vi "Exporting.vi"() -> ()   [LabVIEW 2010]
uses:
  C:/BaseI/CodeBase/Applications/Assemblies/Spiricon.BeamGage.Automation.Interfaces.dll
  Applications/Assemblies/Spiricon.BeamGage.Automation.Interfaces.dll
  C:/BaseI/CodeBase/Applications/Assemblies/Spiricon.BeamGage.Automation.dll
  Applications/Assemblies/Spiricon.BeamGage.Automation.dll
panel:
  out "event callback refnum":refnum<k27>
  in  "FramesPerSec":dbl
  in  "FrameBuffer":dbl
  out "2D Picture":picture
  out "Callback2Exists":bool
  out "Callback1Exists":bool
  in  "STOP SERVER":bool
  in  "START_STOP":bool
  out "AExportStatusEnum":T1(ring)
  in  "EXPORT IMAGE":bool
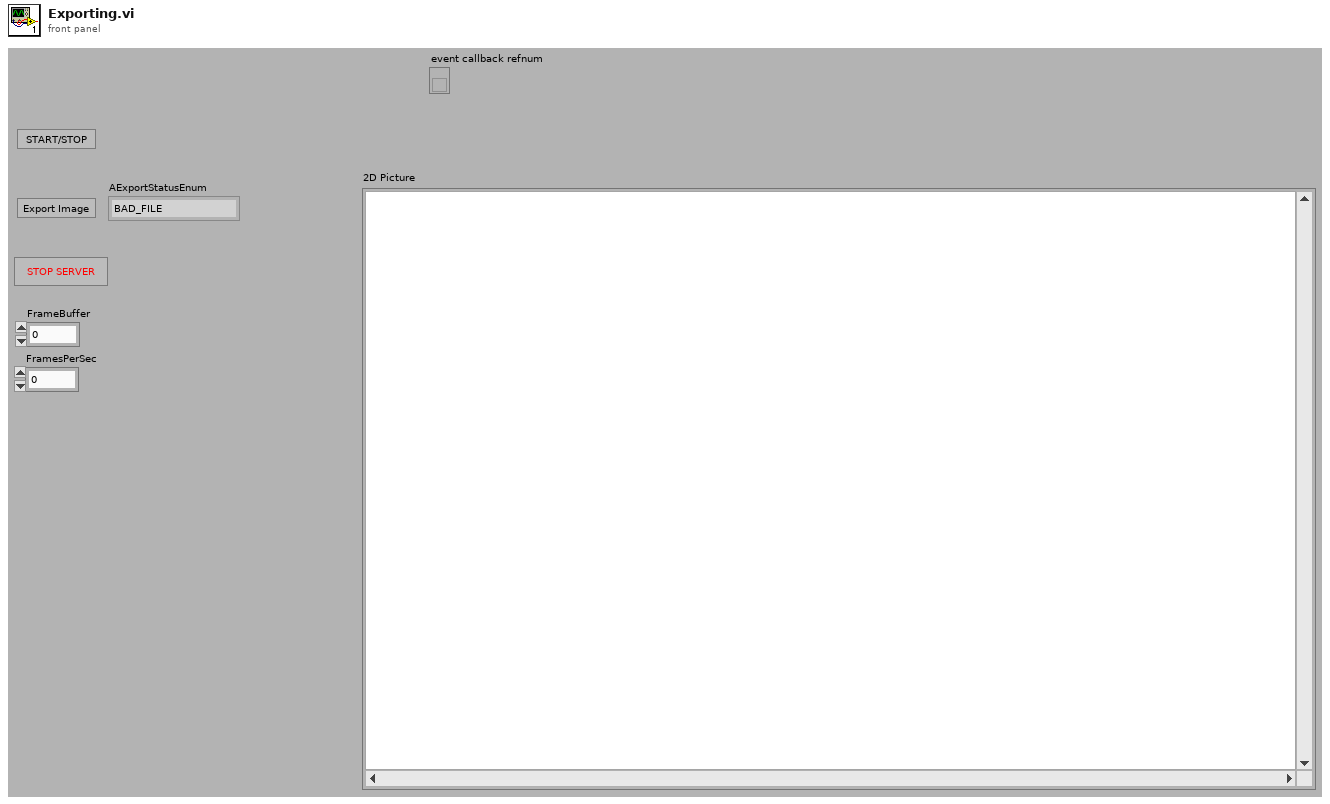
[diagram p1: front panel]
types:
  T1 = enum16{"BAD_FILE", "BAD_FRAME_NUM", "BASE_FILE_EXISTS", "BASE_FILE_IS_DIRECTORY", "GOOD", "NO_FILE_NAME", "NO_IMAGE", "READ_ONLY", "null"}
  T2 = cluster{"FrameBuffer":refnum<vi>, "2D Picture":refnum<vi>, "GetV5Instance":refnum<k24>, "FramesPerSec":refnum<vi>}
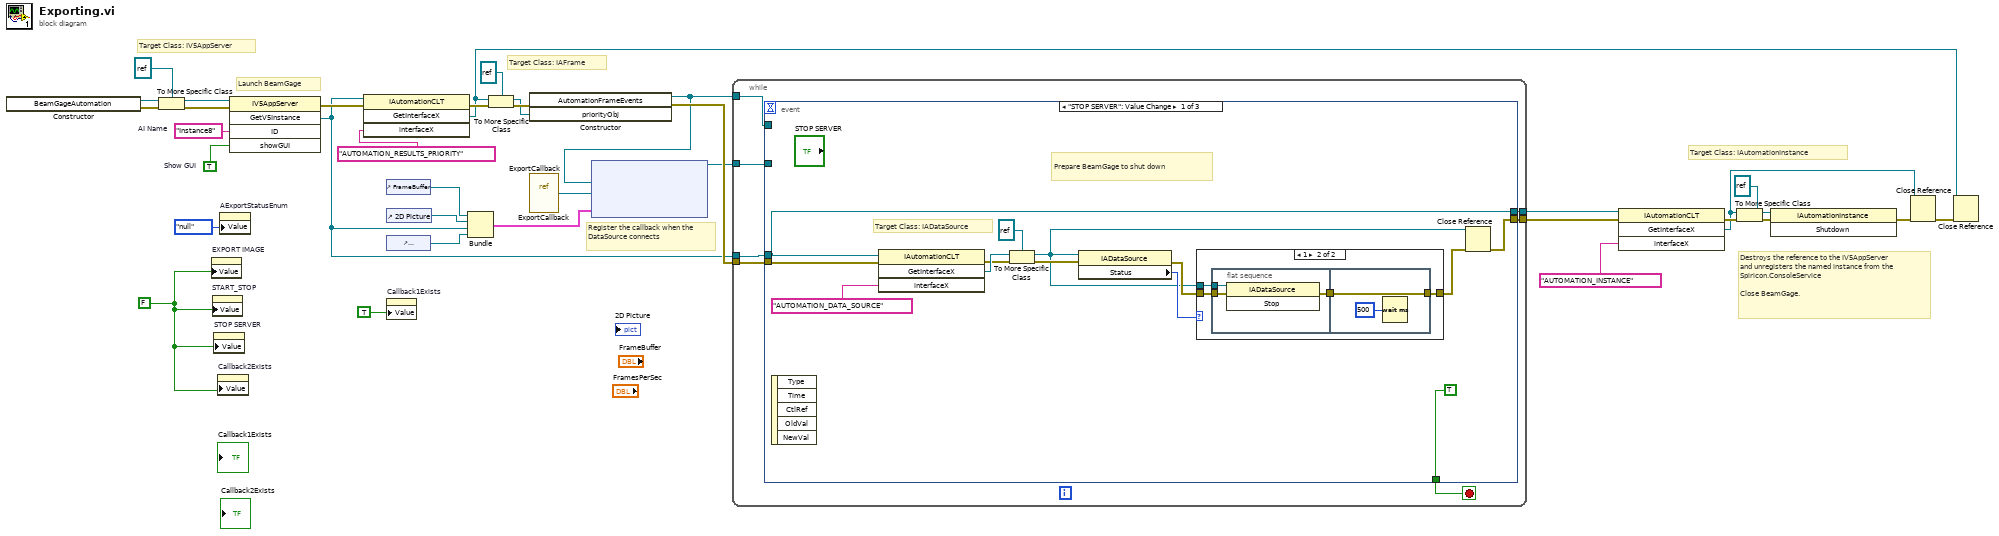
[diagram p0: block diagram]
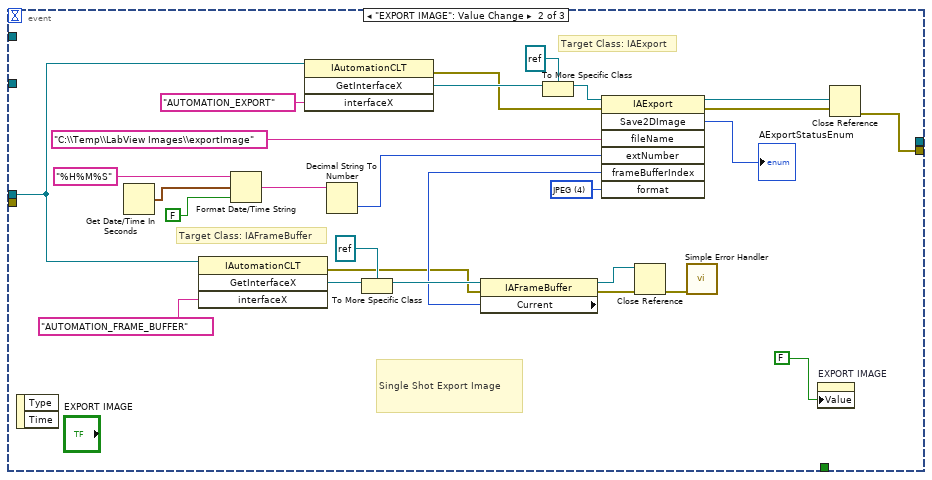
[diagram p3: hidden frame]
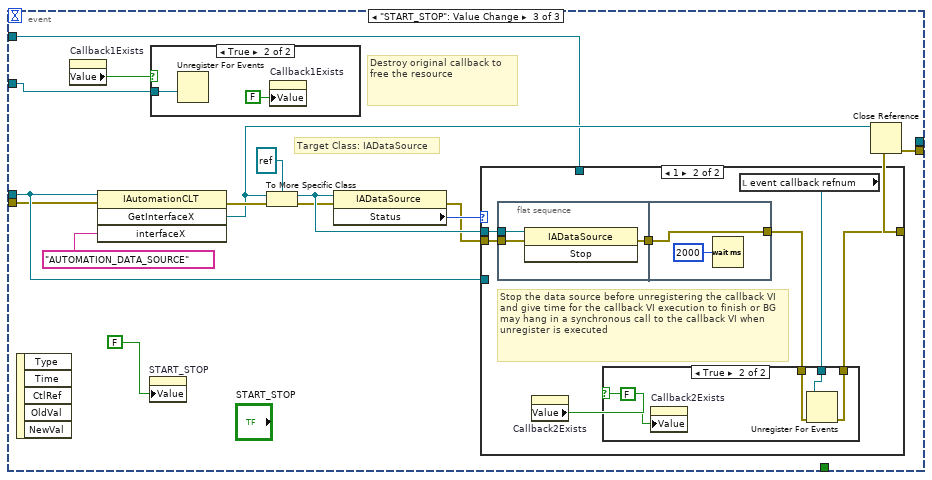
[diagram p4: hidden frame]
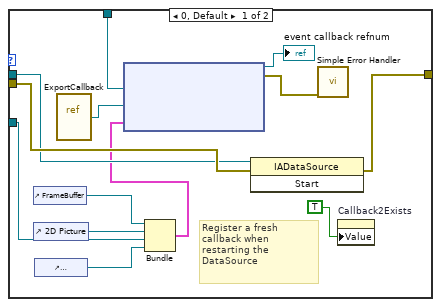
[diagram p6: hidden frame]
diagram:
  w24 = TRUE  # Show GUI
  w28 = "Instance8"  # AI Name
  w9 = FALSE ("stop")
  # "Register the callback when the DataSource connects"
  # "Launch BeamGage"
  # "Target Class: IAFrame"
  # "Target Class: IV5AppServer"
  # "Destroys the reference to the IV5AppServer and unregisters the named instance from the Spiricon.ConsoleService\n\nClose BeamGage."
  # "Target Class: IAutomationInstance"
  n1 = constructor class="BeamGageAutomation"() -> (reference out=w25:refnum<k24>, error out=w32:errorcluster)  [unwired: 3 in, 1 out]
  n2 = To More Specific Class(target class=refnum<k24> refnum, reference=w25, error in=w32) -> (specific class reference=w30:refnum<k24>, error out=w31:errorcluster)
  n3 = property on="EXPORT IMAGE" class="Bool (strict)"("Value"=w9) -> ()  [unwired: 2 in, 2 out]
  n4 = property on="START_STOP" class="Bool (strict)"("Value"=w9) -> ()  [unwired: 2 in, 2 out]
  n5 = property on="STOP SERVER" class="Bool (strict)"("Value"=w9) -> ()  [unwired: 2 in, 2 out]
  n6 = property on="Callback2Exists" class="Bool (strict)"("Value"=w9) -> ()  [unwired: 2 in, 2 out]
  n7 = property on="AExportStatusEnum" class="Enum (strict)"("Value"=T1."null" ("AExportStatusEnum")) -> ()  [unwired: 2 in, 2 out]
  n8 = invoke class="IV5AppServer" method="GetV5Instance"(reference=w30, error in=w31, "ID"=w28, "showGUI"=w24) -> (error out=w29:errorcluster, "GetV5Instance"=w5:refnum<k24>)  [unwired: 1 in, 3 out]
  n9 = invoke class="IAutomationCLT" method="GetInterfaceX"(reference=w5, error in=w29, "interfaceX"="AUTOMATION_RESULTS_PRIORITY") -> (error out=w35:errorcluster, "GetInterfaceX"=w7:refnum<k24>)  [unwired: 1 in, 2 out]
  n10 = control-ref of="FrameBuffer"() -> (w4:refnum<vi>)
  n11 = control-ref of="2D Picture"() -> (w6:refnum<vi>)
  n12 = control-ref of="FramesPerSec"() -> (w2:refnum<vi>)
  n13 = property on="Callback1Exists" class="Bool (strict)"("Value"=TRUE ("CallbackExists")) -> ()  [unwired: 2 in, 2 out]
  n14 = Bundle("FrameBuffer"=w4, "2D Picture"=w6, "GetV5Instance"=w5, "FramesPerSec"=w2) -> (w1:T2)  [unwired: 1 in]
  n15 = To More Specific Class(target class=refnum<k24> refnum, reference=w7, error in=w35) -> (specific class reference=w26:refnum<k24>, error out=w36:errorcluster)
  n16 = constructor class="AutomationFrameEvents"(error in=w36, "priorityObj"=w26) -> (reference out=w11:refnum<k24>, error out=w14:errorcluster)  [unwired: 2 in, 2 out]
  n17 = vi-ref "ExportCallback.vi"() -> ("vi reference"=w3:refnum<vi>)
  n18 = vi-ref "ExportCallback.vi"() -> ()  [unwired: 1 out]
  n19 = node(w11, w3, w1) -> (w12:refnum<k27>)  [unwired: 2 in, 1 out]
  n20 = while {
    tunnel: [w43] -> w16
    tunnel: w5 -> [w39]
    tunnel: w14 -> [w41]
    tunnel: [w40] -> w15
    tunnel: w11 -> [w38]
    tunnel: w12 -> [w37]
    stop <- w42 stop-if-true
    n21 = event shown="[0] \"STOP SERVER\": Value Change" {
      selector: _ -> [_ _ _]
      dyn-events: _ -> [_ _ _]
      timeout: _ -> [_ _ _]
      tunnel: [w44 _ _] -> w43
      tunnel: [TRUE ("stop") _ _] -> w42
      tunnel: w41 -> [w47 _ w96]
      tunnel: [w48 w70 w97] -> w40
      tunnel: w39 -> [w44 w73 w98]
      tunnel: w38 -> [_ _ w99]
      tunnel: w37 -> [_ _ w95]
      event "STOP SERVER": Value Change {
        # "Prepare BeamGage to shut down"
        # "Target Class: IADataSource"
        n22 = event-data() -> ()  [unwired: 1 in, 5 out]
        n23 = invoke class="IAutomationCLT" method="GetInterfaceX"(reference=w44, error in=w47, "interfaceX"="AUTOMATION_DATA_SOURCE") -> (error out=w52:errorcluster, "GetInterfaceX"=w55:refnum<k24>)  [unwired: 1 in, 2 out]
        n24 = To More Specific Class(target class=refnum<k24> refnum, reference=w55, error in=w52) -> (specific class reference=w45:refnum<k24>, error out=w50:errorcluster)
        n25 = property class="IADataSource"(reference=w45, error in=w50) -> (error out=w53:errorcluster, "Status"=w49:i32)  [unwired: 1 out]
        n26 = case shown="1" w49 {
          tunnel: w45 -> [_ w61]
          tunnel: w53 -> [w57 w60]
          tunnel: [w57 w59] -> w54
          frame 0, Default {
          }
          frame 1 {
            n27 = flat-sequence {
              tunnel: w61 -> [w64]
              tunnel: w60 -> [w63]
              tunnel: [w62] -> w58
              tunnel: [w65] -> w59
              tunnel: w58 -> [w65]
              frame #0 {
                n28 = invoke class="IADataSource" method="Stop"(reference=w64, error in=w63) -> (error out=w62:errorcluster)  [unwired: 1 in, 2 out]
              }
              frame #1 {
                n29 = Wait (ms)(milliseconds to wait=u32 500) -> ()  [unwired: 1 out]
              }
            }
          }
        }
        n30 = Close Reference(reference=w45, error in (no error)=w54) -> (error out=w48:errorcluster)
      }
      event "EXPORT IMAGE": Value Change {
        w84 = 4 items=["NONE", "ASCII", "BMP", "GIF", "JPEG", "PNG", "TIFF"] ("format")
        # "Single Shot Export Image"
        # "Target Class: IAFrameBuffer"
        # "Target Class: IAExport"
        n31 = event-data() -> ()  [unwired: 1 in, 2 out]
        n32 = Get Date/Time In Seconds() -> (seconds since 1Jan1904=w91:timestamp)
        n33 = invoke class="IAutomationCLT" method="GetInterfaceX"(reference=w73, "interfaceX"="AUTOMATION_FRAME_BUFFER") -> (error out=w71:errorcluster, "GetInterfaceX"=w78:refnum<k24>)  [unwired: 2 in, 2 out]
        n34 = Format Date/Time String(time format string (%c)="%H%M%S", seconds (now)=w91, UTC format=FALSE) -> (date/time string=w87:string)
        n35 = invoke class="IAutomationCLT" method="GetInterfaceX"(reference=w73, "interfaceX"="AUTOMATION_EXPORT") -> (error out=w72:errorcluster, "GetInterfaceX"=w81:refnum<k24>)  [unwired: 2 in, 2 out]
        n36 = Decimal String To Number(string=w87) -> (number=w88:i32)  [unwired: 2 in, 1 out]
        n37 = To More Specific Class(target class=refnum<k24> refnum, reference=w78) -> (specific class reference=w76:refnum<k24>)  [unwired: 1 in, 1 out]
        n38 = property class="IAFrameBuffer"(reference=w76, error in=w71) -> (reference out=w67:refnum<k24>, error out=w68:errorcluster, "Current"=w75:u32)
        n39 = To More Specific Class(target class=refnum<k24> refnum, reference=w81) -> (specific class reference=w92:refnum<k24>)  [unwired: 1 in, 1 out]
        n40 = invoke class="IAExport" method="Save2DImage"(reference=w92, error in=w72, "fileName"="C:\\Temp\\LabView Images\\exportImage", "extNumber"=w88, "frameBufferIndex"=w75, "format"=w84) -> (reference out=w86:refnum<k24>, error out=w85:errorcluster, "Save2DImage"=→"AExportStatusEnum":i32)  [unwired: 1 in, 4 out]
        n41 = Close Reference(reference=w67, error in (no error)=w68) -> (error out=w69:errorcluster)
        n42 = call <vilib>:"Simple Error Handler.vi"("error in (no error)"=w69) -> ()  [unwired: 4 in, 5 out]
        n43 = property on="EXPORT IMAGE" class="Bool (strict)"("Value"=FALSE ("stop")) -> ()  [unwired: 2 in, 2 out]
        n44 = Close Reference(reference=w86, error in (no error)=w85) -> (error out=w70:errorcluster)
      }
      event "START_STOP": Value Change {
        # "Destroy original callback to free the resource"
        # "Target Class: IADataSource"
        n45 = event-data() -> ()  [unwired: 1 in, 5 out]
        n46 = property on="Callback1Exists" class="Bool (strict)"() -> ("Value"=w94:bool)  [unwired: 2 in, 2 out]
        n47 = invoke class="IAutomationCLT" method="GetInterfaceX"(reference=w98, error in=w96, "interfaceX"="AUTOMATION_DATA_SOURCE") -> (error out=w104:errorcluster, "GetInterfaceX"=w100:refnum<k24>)  [unwired: 1 in, 2 out]
        n48 = property on="START_STOP" class="Bool (strict)"("Value"=FALSE ("stop")) -> ()  [unwired: 2 in, 2 out]
        n49 = case shown="True" w94 {
          tunnel: w95 -> [_ w111]
          frame False {
          }
          frame True {
            n50 = Unregister For Events(event registration refnum=w111) -> ()  [unwired: 1 in, 1 out]
            n51 = property on="Callback1Exists" class="Bool (strict)"("Value"=FALSE ("CallbackExists")) -> ()  [unwired: 2 in, 2 out]
          }
        }
        n52 = To More Specific Class(target class=refnum<k24> refnum, reference=w100, error in=w104) -> (specific class reference=w109:refnum<k24>, error out=w107:errorcluster)
        n53 = property class="IADataSource"(reference=w109, error in=w107) -> (error out=w103:errorcluster, "Status"=w108:i32)  [unwired: 1 out]
        n54 = case shown="1" w108 {
          tunnel: w109 -> [w119 w130]
          tunnel: w103 -> [w121 w129]
          tunnel: [w124 w127] -> w101
          tunnel: w99 -> [w123 _]
          tunnel: w98 -> [w117 _]
          frame 0, Default {
            # "Register a fresh callback when restarting the DataSource"
            n55 = control-ref of="FrameBuffer"() -> (w118:refnum<vi>)
            n56 = control-ref of="2D Picture"() -> (w120:refnum<vi>)
            n57 = control-ref of="FramesPerSec"() -> (w115:refnum<vi>)
            n58 = vi-ref "ExportCallback.vi"() -> ("vi reference"=w113:refnum<vi>)
            n59 = Bundle("FrameBuffer"=w118, "2D Picture"=w120, "GetV5Instance"=w117, "FramesPerSec"=w115) -> (w112:T2)  [unwired: 1 in]
            n60 = node(w123, w113, w112) -> (→"event callback refnum":refnum<k27>, w122:errorcluster)  [unwired: 2 in]
            n61 = invoke class="IADataSource" method="Start"(reference=w119, error in=w121) -> (error out=w124:errorcluster)  [unwired: 1 in, 2 out]
            n62 = call <vilib>:"Simple Error Handler.vi"("error in (no error)"=w122) -> ()  [unwired: 4 in, 5 out]
            n63 = property on="Callback2Exists" class="Bool (strict)"("Value"=TRUE ("CallbackExists")) -> ()  [unwired: 2 in, 2 out]
          }
          frame 1 {
            # "Stop the data source before unregistering the callback VI  and give time for the callback VI execution to finish or BG may hang in a synchronous call to the callback VI when unregister is executed"
            n64 = flat-sequence {
              tunnel: w130 -> [w138]
              tunnel: w129 -> [w137]
              tunnel: [w136] -> w131
              tunnel: [w139] -> w128
              tunnel: w131 -> [w139]
              frame #0 {
                n65 = invoke class="IADataSource" method="Stop"(reference=w138, error in=w137) -> (error out=w136:errorcluster)  [unwired: 1 in, 2 out]
              }
              frame #1 {
                n66 = Wait (ms)(milliseconds to wait=u32 2000) -> ()  [unwired: 1 out]
              }
            }
            n67 = property on="Callback2Exists" class="Bool (strict)"() -> ("Value"=w126:bool)  [unwired: 2 in, 2 out]
            n68 = local read "event callback refnum"() -> (w125:refnum<k27>)
            n69 = case shown="True" w126 {
              tunnel: w125 -> [_ w135]
              tunnel: w128 -> [_ w133]
              tunnel: [_ w132] -> w127
              frame False {
              }
              frame True {
                n70 = property on="Callback2Exists" class="Bool (strict)"("Value"=FALSE ("CallbackExists")) -> ()  [unwired: 2 in, 2 out]
                n71 = Unregister For Events(event registration refnum=w135, error in=w133) -> (error out=w132:errorcluster)
              }
            }
          }
        }
        n72 = Close Reference(reference=w100, error in (no error)=w101) -> (error out=w97:errorcluster)
      }
    }
  }
  n73 = invoke class="IAutomationCLT" method="GetInterfaceX"(reference=w16, error in=w15, "interfaceX"="AUTOMATION_INSTANCE") -> (error out=w19:errorcluster, "GetInterfaceX"=w17:refnum<k24>)  [unwired: 1 in, 2 out]
  n74 = To More Specific Class(target class=refnum<k24> refnum, reference=w17, error in=w19) -> (specific class reference=w20:refnum<k24>, error out=w18:errorcluster)
  n75 = invoke class="IAutomationInstance" method="Shutdown"(reference=w20, error in=w18) -> (error out=w23:errorcluster)  [unwired: 1 in, 2 out]
  n76 = Close Reference(reference=w17, error in (no error)=w23) -> (error out=w8:errorcluster)
  n77 = Close Reference(reference=w7, error in (no error)=w8) -> ()  [unwired: 1 out]
